vi "Peregrine_set_motor_parameters.vi"(0 "Handle in":refnum<visa-resource-name>, 2 "Address":u8, 5 "Select parameter":T1(ring), 9 "Value":dbl, 11 "error":errorcluster) -> (4 "Handle out":refnum<visa-resource-name>, 6 "Key response":u32, 8 "Raw value response":i32, 10 "Decoded value response":dbl, 15 "error out":errorcluster)   [LabVIEW 2019]
panel:
  # "Inputs"
  # "Response message"
  # "Output"
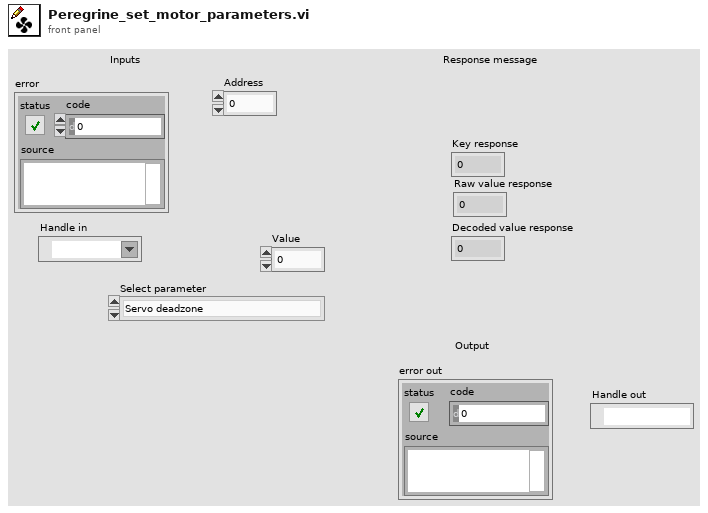
[diagram p1: front panel]
types:
  T1 = enum16{"Servo deadzone", "Position target gain", "Position target P", "Position target D", "V target P", "V target D", "Frequency slew", "Motor direction", "Error gain", "LQR K0", "LQR K1", "LQR B1", "Encoder DIV", "FDIR steprate"}
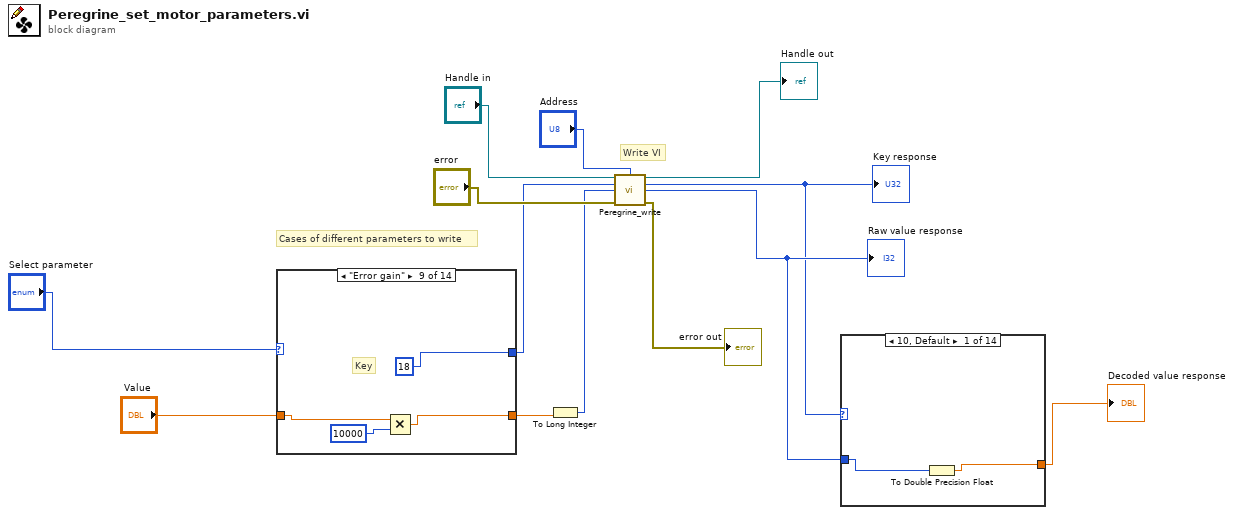
[diagram p0: block diagram]
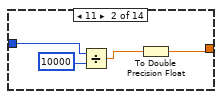
[diagram p2: hidden frame]
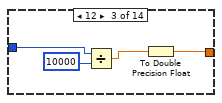
[diagram p3: hidden frame]
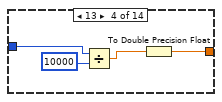
[diagram p4: hidden frame]
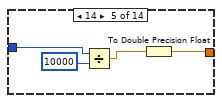
[diagram p5: hidden frame]
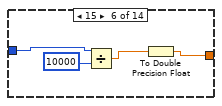
[diagram p6: hidden frame]
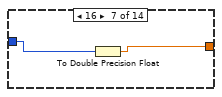
[diagram p7: hidden frame]
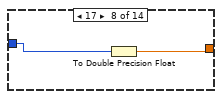
[diagram p8: hidden frame]
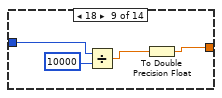
[diagram p9: hidden frame]
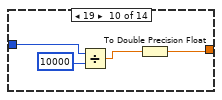
[diagram p10: hidden frame]
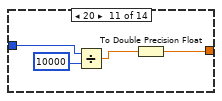
[diagram p11: hidden frame]
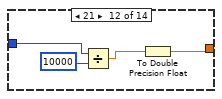
[diagram p12: hidden frame]
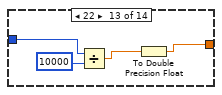
[diagram p13: hidden frame]
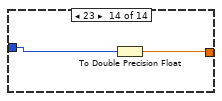
[diagram p14: hidden frame]
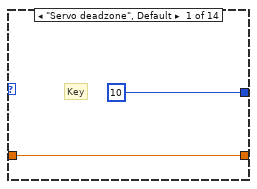
[diagram p15: hidden frame]
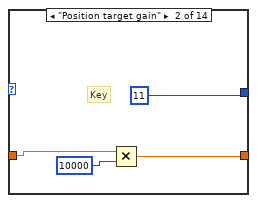
[diagram p16: hidden frame]
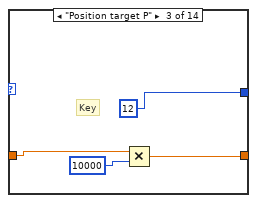
[diagram p17: hidden frame]
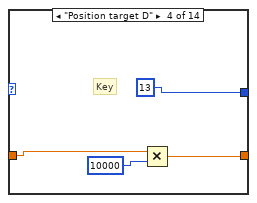
[diagram p18: hidden frame]
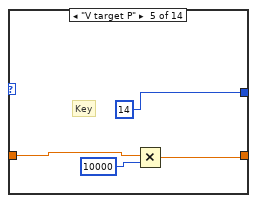
[diagram p19: hidden frame]
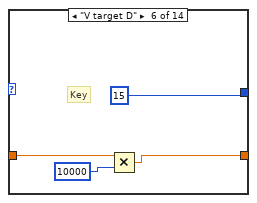
[diagram p20: hidden frame]
diagram:
  # "Cases of different parameters to write"
  # "Write VI"
  n1 = case shown="\"Error gain\"" "Select parameter" {
    tunnel: [u32 10 u32 11 u32 12 u32 13 u32 14 u32 15 u32 16 u32 17 u32 18 u32 19 u32 20 u32 21 u32 22 u32 23] -> w6
    tunnel: "Value" -> [w14 w18 w22 w26 w29 w33 w36 w38 w42 w46 w49 w53 w57 w60]
    tunnel: [w14 w16 w20 w24 w28 w32 w36 w38 w40 w44 w48 w52 w56 w60] -> w10
    frame "Servo deadzone", Default {
      # "Key"
    }
    frame "Position target gain" {
      # "Key"
      n2 = Multiply(x=w18, y=10000) -> (x*y=w16:dbl)
    }
    frame "Position target P" {
      # "Key"
      n3 = Multiply(x=w22, y=10000) -> (x*y=w20:dbl)
    }
    frame "Position target D" {
      # "Key"
      n4 = Multiply(x=w26, y=10000) -> (x*y=w24:dbl)
    }
    frame "V target P" {
      # "Key"
      n5 = Multiply(x=w29, y=10000) -> (x*y=w28:dbl)
    }
    frame "V target D" {
      # "Key"
      n6 = Multiply(x=w33, y=10000) -> (x*y=w32:dbl)
    }
    frame "Frequency slew" {
      # "Key"
    }
    frame "Motor direction" {
      # "Key"
    }
    frame "Error gain" {
      # "Key"
      n7 = Multiply(x=w42, y=10000) -> (x*y=w40:dbl)
    }
    frame "LQR K0" {
      # "Key"
      n8 = Multiply(x=w46, y=10000) -> (x*y=w44:dbl)
    }
    frame "LQR K1" {
      # "Key"
      n9 = Multiply(x=w49, y=10000) -> (x*y=w48:dbl)
    }
    frame "LQR B1" {
      # "Key"
      n10 = Multiply(x=w53, y=10000) -> (x*y=w52:dbl)
    }
    frame "Encoder DIV" {
      # "Key"
      n11 = Multiply(x=w57, y=10000) -> (x*y=w56:dbl)
    }
    frame "FDIR steprate" {
      # "Key"
    }
  }
  n12 = To Long Integer(number=w10) -> (32bit integer=w5:i32)
  n13 = call "Peregrine_write.vi"("Handle in"="Handle in", "Address"="Address", "Key"=w6, "Value"=w5, "error"="error") -> ("Handle out"=→"Handle out":refnum<visa-resource-name>, "Key response"=w1:u32, "Value response"=w2:i32, "error out"=→"error out":errorcluster)  [unwired: 7 in]
  "Key response" <- w1
  "Raw value response" <- w2
  n14 = case shown="10, Default" w1 {
    tunnel: [w63 w65 w69 w73 w77 w81 w85 w87 w89 w93 w97 w101 w105 w109] -> w11
    tunnel: w2 -> [w62 w64 w68 w72 w76 w80 w84 w86 w88 w92 w96 w100 w104 w108]
    frame 10, Default {
      n15 = To Double Precision Float(number=w62) -> (double precision float=w63:dbl)
    }
    frame 11 {
      n16 = Divide(x=w64, y=10000) -> (x/y=w66:dbl)
      n17 = To Double Precision Float(number=w66) -> (double precision float=w65:dbl)
    }
    frame 12 {
      n18 = Divide(x=w68, y=10000) -> (x/y=w70:dbl)
      n19 = To Double Precision Float(number=w70) -> (double precision float=w69:dbl)
    }
    frame 13 {
      n20 = Divide(x=w72, y=10000) -> (x/y=w74:dbl)
      n21 = To Double Precision Float(number=w74) -> (double precision float=w73:dbl)
    }
    frame 14 {
      n22 = Divide(x=w76, y=10000) -> (x/y=w78:dbl)
      n23 = To Double Precision Float(number=w78) -> (double precision float=w77:dbl)
    }
    frame 15 {
      n24 = Divide(x=w80, y=10000) -> (x/y=w82:dbl)
      n25 = To Double Precision Float(number=w82) -> (double precision float=w81:dbl)
    }
    frame 16 {
      n26 = To Double Precision Float(number=w84) -> (double precision float=w85:dbl)
    }
    frame 17 {
      n27 = To Double Precision Float(number=w86) -> (double precision float=w87:dbl)
    }
    frame 18 {
      n28 = Divide(x=w88, y=10000) -> (x/y=w90:dbl)
      n29 = To Double Precision Float(number=w90) -> (double precision float=w89:dbl)
    }
    frame 19 {
      n30 = Divide(x=w92, y=10000) -> (x/y=w94:dbl)
      n31 = To Double Precision Float(number=w94) -> (double precision float=w93:dbl)
    }
    frame 20 {
      n32 = Divide(x=w96, y=10000) -> (x/y=w98:dbl)
      n33 = To Double Precision Float(number=w98) -> (double precision float=w97:dbl)
    }
    frame 21 {
      n34 = Divide(x=w100, y=10000) -> (x/y=w102:dbl)
      n35 = To Double Precision Float(number=w102) -> (double precision float=w101:dbl)
    }
    frame 22 {
      n36 = Divide(x=w104, y=10000) -> (x/y=w106:dbl)
      n37 = To Double Precision Float(number=w106) -> (double precision float=w105:dbl)
    }
    frame 23 {
      n38 = To Double Precision Float(number=w108) -> (double precision float=w109:dbl)
    }
  }
  "Decoded value response" <- w11
